vi "L21.vi"() -> ()   [LabVIEW 2014]
panel:
  in  "L21":dbl
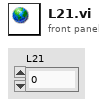
[diagram p1: front panel]
diagram:
